vi "TSCAN Demo TC1001.vi"() -> ()   [LabVIEW 2013]
uses:
  TSCAN Dll.vi
  TSCAN Init.vi
  TSCAN ChannelCount.vi
  TSCAN SetMapping.vi
  TSCAN LoadDBC.vi
  TSCAN Open.vi
  TSCAN Close.vi
panel:
  out "Connect_TSCAN_Successfully":bool
  out "DBC Data":T1 {"ID" format="%x"}
  in  "ADBCAbsolutePath":path=path "C:/Users/DYR/Desktop/M110.dbc"
  in  "Tsapp_set_mapping_verbose_Type":T2={"AAppChannelType"=0, "AAppChannel"=0, "AHardwareType"=3, "AHardwareSubType"=3, "HardwareIndex"=0, "AHardwareChannel"=0, "AEnableMapping"=1, "ABaudrateKbps"=500.0, "AListenOnly"=0, "Int120Ohm"=1} {"Int120Ohm" items=["Disable", "Enable"]; "AListenOnly" items=["Normal", "ListenOnly"]; "ABaudrateKbps" format="%#_g  k"; "AEnableMapping" items=["Disable", "Enable"]; "AAppChannelType" items=["APP_CAN", "APP_LIN"]; "AHardwareChannel" items=["CHN1", "CHN2", "CHN3", "CHN4", "CHN5", "CHN6", "CHN7", "CHN8", "CHN9", "CHN10", "CHN11", "CHN12", "CHN13", "CHN14", "CHN15", "CHN16", "CHN17", "CHN18", "CHN19", "CHN20", "CHN21", "CHN22", "CHN23", "CHN24", "CHN25", "CHN26", "CHN27", "CHN28", "CHN29", "CHN30", "CHN31", "CHN32"]; "AAppChannel" items=["CHN1", "CHN2", "CHN3", "CHN4", "CHN5", "CHN6", "CHN7", "CHN8", "CHN9", "CHN10", "CHN11", "CHN12", "CHN13", "CHN14", "CHN15", "CHN16", "CHN17", "CHN18", "CHN19", "CHN20", "CHN21", "CHN22", "CHN23", "CHN24", "CHN25", "CHN26", "CHN27", "CHN28", "CHN29", "CHN30", "CHN31", "CHN32"]; "AHardwareType" items=["BUS_UNKNOWN_TYPE", "TS_TCP_DEVICE", "XL_USB_DEVICE", "TS_USB_DEVICE", "PEAK_USB_DEVICE", "KVASER_USB_DEVICE", "ZLG_USB_DEVICE", "ICS_USB_DEVICE", "TS_TC1005_DEVICE"]; "AHardwareSubType" items=["TS_UNKNOWN_DEVICE", "TSCAN_PRO", "TSCAN_Litel", "TC1001", "TL1001", "TC1011", "TSInterface", "TC1002", "TC1014"]}
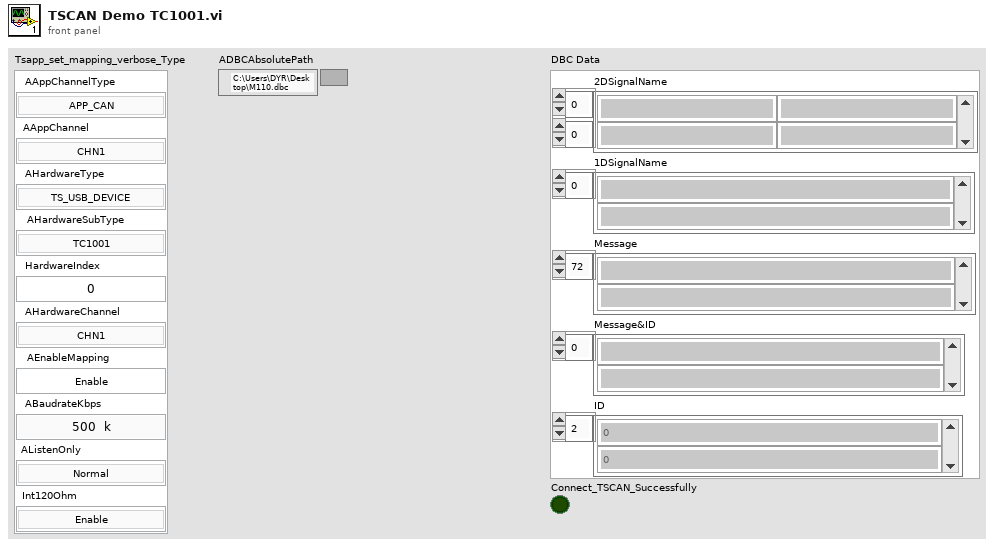
[diagram p1: front panel]
types:
  T1 = cluster{"2DSignalName":string[][], "1DSignalName":string[], "Message":string[], "Message&ID":string[], "ID":i32[]}
  T2 = cluster{"AAppChannelType":i32, "AAppChannel":i32, "AHardwareType":i32, "AHardwareSubType":i32, "HardwareIndex":i32, "AHardwareChannel":i32, "AEnableMapping":u32, "ABaudrateKbps":sgl, "AListenOnly":u32, "Int120Ohm":u32}
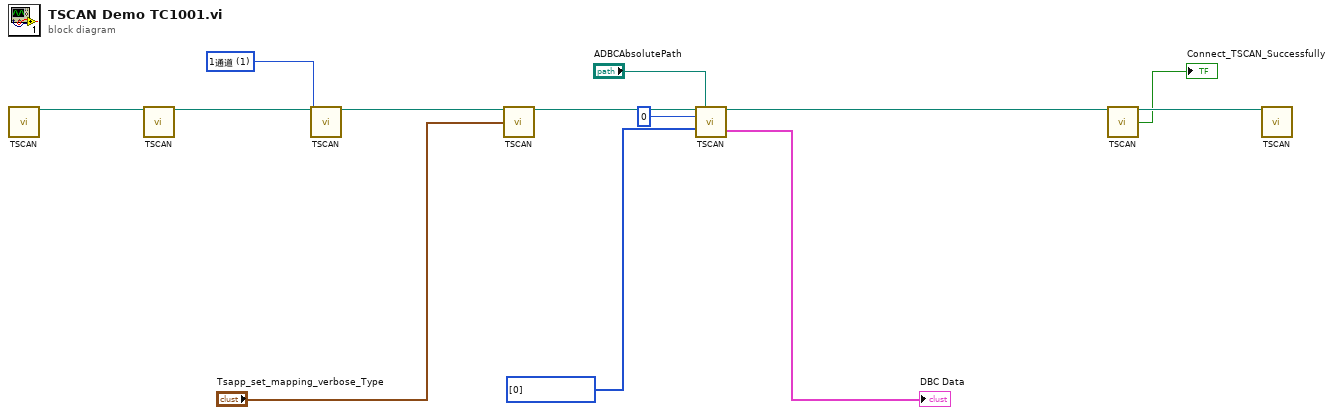
[diagram p0: block diagram]
diagram:
  w6 = i32[] [0] items=["CHN1", "CHN2", "CHN3", "CHN4", "CHN5", "CHN6", "CHN7", "CHN8", "CHN9", "CHN10", "CHN11", "CHN12", "CHN13", "CHN14", "CHN15", "CHN16", "CHN17", "CHN18", "CHN19", "CHN20", "CHN21", "CHN22", "CHN23", "CHN24", "CHN25", "CHN26", "CHN27", "CHN28", "CHN29", "CHN30", "CHN31", "CHN32"] ("ABindChannels")
  w11 = 1 items=["1通道"=1, "2通道"=2, "3通道"=3, "4通道"=4, "5通道"=5] ("使用通道数量")
  n1 = call-poly "TSCAN.vi"() -> ("DllPath"=w13:path)  [unwired: 15 in]
  n2 = call-poly "TSCAN.vi"("路径输入"=w13) -> ("路径输出"=w12:path)  [unwired: 13 in, 1 out]
  n3 = call-poly "TSCAN.vi"("路径输入"=w12, "使用通道数量"=w11) -> ("路径输出"=w10:path)  [unwired: 11 in, 2 out]
  n4 = call-poly "TSCAN.vi"("路径输入"=w10, "Tsapp_set_mapping_verbose_Type"="Tsapp_set_mapping_verbose_Type") -> ("路径输出"=w8:path)  [unwired: 12 in, 1 out]
  n5 = call-poly "TSCAN.vi"("路径输入"=w8, "ADBCAbsolutePath"="ADBCAbsolutePath", "AIdIn"=0, "ABindChannels"=w6) -> ("路径输出"=w3:path, "DBC Data"=→"DBC Data":T1)  [unwired: 8 in, 2 out]
  n6 = call-poly "TSCAN.vi"("路径输入"=w3) -> ("路径输出"=w2:path, "Connect_TSCAN_Successfully"=→"Connect_TSCAN_Successfully":bool)  [unwired: 12 in, 1 out]
  n7 = call-poly "TSCAN.vi"("路径输入"=w2) -> ()  [unwired: 13 in, 2 out]
